vi "Write Status_Ref.vi"(8 "error in (no error)":errorcluster, 10 "Status_Ref":refnum<vi>, 11 "PowerSupply in":refnum<class "PowerSupply.lvclass">) -> (0 "error out":errorcluster, 3 "PowerSupply out":refnum<class "PowerSupply.lvclass">)   [LabVIEW 2019, in "PowerSupply.lvlib" / "PowerSupply.lvclass"]
uses:
  Library/PowerSupply.lvclass
  Custom Controls/Status_Flags.ctl
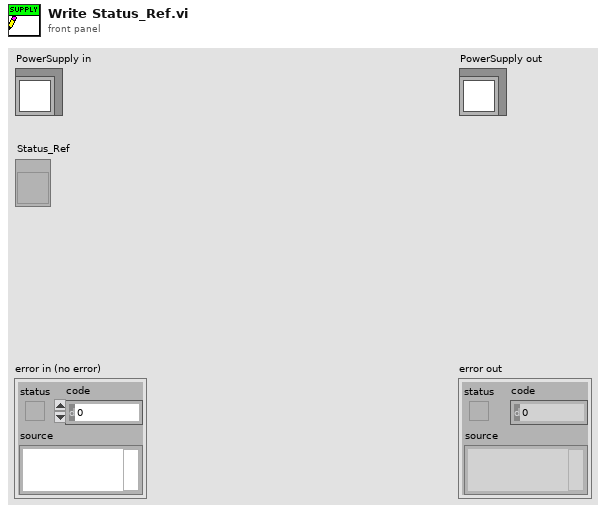
[diagram p1: front panel]
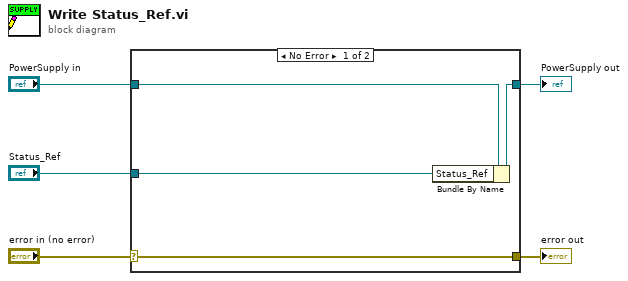
[diagram p0: block diagram]
diagram:
  n1 = case shown="No Error" "error in (no error)" {
    selector: "error in (no error)" -> [w9 w10]
    tunnel: [w9 w10] -> w4
    tunnel: [w7 w11] -> w2
    tunnel: "PowerSupply in" -> [w8 w11]
    tunnel: "Status_Ref" -> [w6 _]
    frame No Error {
      n2 = Bundle By Name(cluster=w8, "Status_Ref"=w6) -> (w7:refnum<class "PowerSupply.lvclass">)
    }
    frame Error {
    }
  }
  "error out" <- w4
  "PowerSupply out" <- w2
